vi "AutoScroll Read.vi"(4 "error in (no error)":errorcluster, 6 "Container State":T3, 7 "Display State In":T1={"logTable"=refnum, "max items"=500, "displaydata"=[], "data"=[], "Auto Scroll"=TRUE, "current item"=500, "col headers"=[], "Add to Top"=TRUE, "Auto resize"=TRUE, "col size"=[], "filters"=[], "color cells"=[]}) -> (0 "error out":errorcluster, 2 "Value":bool, 3 "Display State Out":T1={"logTable"=refnum, "max items"=500, "displaydata"=[], "data"=[], "Auto Scroll"=TRUE, "current item"=500, "col headers"=[], "Add to Top"=TRUE, "Auto resize"=TRUE, "col size"=[], "filters"=[], "color cells"=[]})   [LabVIEW 2013, in "UI-DisplayTable(dev).xctl"]
uses:
  UI-DisplayTable(dev).xctl
  <vilib>/_xctls/Container State.ctl
  State.ctl
  Support/DEF-Filter.ctl
  <vilib>/_xctls/XControlSupport.lvlib
panel:
  # "Replace the Value Indicator below with an Indicator of desired type.\nDo not remove this Indicator or the others from the connector pane. \nDo not change the connector pane pattern.\nThe Value Indicator should always be the second terminal from top on the output side in the connector pane."
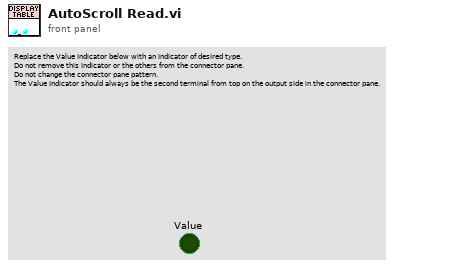
[diagram p1: front panel]
types:
  T1 = typedef "UI-DisplayTable(dev).xctl/State.ctl" = cluster{"logTable":refnum<vi>, "max items":i32, "displaydata":string[][], "data":string[][], "Auto Scroll":bool, "current item":i32, "col headers":string[], "Add to Top":bool, "Auto resize":bool, "col size":i32[], "filters":T2[], "color cells":cluster{"color cell":cluster{"Column":string, "Value":string, "Highlight Column":string}, "Color Box":u32}[]}
  T2 = typedef "UI-DisplayTable(dev).xctl/DEF-Filter.ctl" = cluster{"column":string, "value":string[]}
  T3 = typedef "XControlSupport.lvlib/Container State.ctl" = cluster{"Indicator?":bool, "Run Mode?":bool, " Refnum":refnum<vi>}
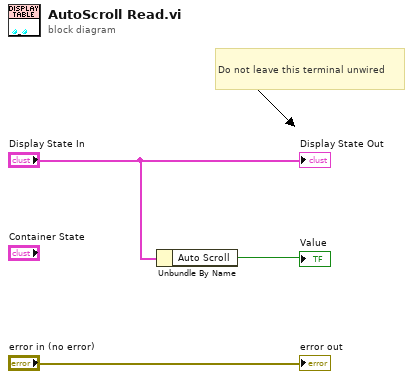
[diagram p0: block diagram]
diagram:
  # "Do not leave this terminal unwired"
  n1 = Unbundle By Name("Display State In") -> ("Auto Scroll"=→"Value":bool)
  "error out" <- "error in (no error)"
  "Display State Out" <- "Display State In"
